vi "GetFPGABitfilePath.vi"(8 "error in (no error)":errorcluster) -> (0 "error out":errorcluster, 2 "description":string, 3 "fpga bitfile":path, 5 "found":bool)   [LabVIEW 2017, in "McsaFpgaBitfileManager.lvlib"]
uses:
  <vilib>/addons/InsightCM/Devices/Shared/Mcsa/McsaFpgaBitfileManager/McsaFpgaBitfileManager.lvlib
  <vilib>/addons/InsightCM/Utilities/GlobalConfiguration/GlobalConfiguration.lvlib
  <vilib>/addons/SystemInfoProcess/SystemInfoProcess.lvlib
  <vilib>/addons/InsightCM/Devices/Shared/Cms/CmsFpgaBitfileManager/CmsFpgaBitfileManager.lvlib
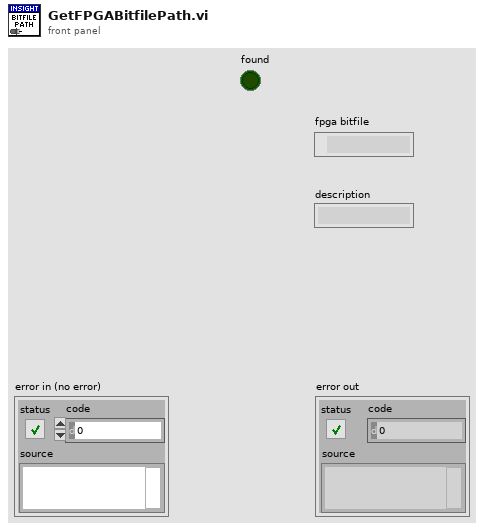
[diagram p1: front panel]
types:
  T1 = typedef "R2_Device.ctl" = cluster{"Id":string, "Name":string, "DeviceType":string, "HardwareName":string, "IpAddress":string, "HardwareInfo":T2[], "ApplicationType":string, "ApplicationVersion":string, "EquipmentIds":string[], "ConfigurationVersion":string, "State":T3, "Properties":T2[], "DataGroups":T4[], "BurstModeTrigger":T8}
  T2 = typedef "KeyValuePair.ctl" = cluster{"Key":string, "Value":string}
  T3 = typedef "DeviceState.ctl" = cluster{"Disabled":bool}
  T4 = typedef "R2_DataGroup.ctl" = cluster{"Name":string, "OperatingStates":T5[], "Properties":T2[], "EquipmentIds":string[], "AssetNodeId":string}
  T5 = typedef "OperatingState.ctl" = cluster{"Name":string, "Properties":T2[], "Triggers":T6[]}
  T6 = typedef "Trigger.ctl" = cluster{"Type":string, "Expression":string, "Conditions":T7[]}
  T7 = typedef "Condition.ctl" = cluster{"Source":string, "Type":string, "Operator":string, "CompareTo":string, "DwellSeconds":dbl}
  T8 = typedef "BurstModeTrigger.ctl" = cluster{"Trigger":T6, "SampleRate":string, "AcquisitionLength":string}
  T9 = typedef "cRIODetectHW.lvlib/SystemHW.ctl" = cluster{"controller":T10, "chassis":T10, "modules":T10[]}
  T10 = typedef "cRIODetectHW.lvlib/cRIO Product Info.ctl" = cluster{"vendorName":string, "productName":string, "serialNumber":string}
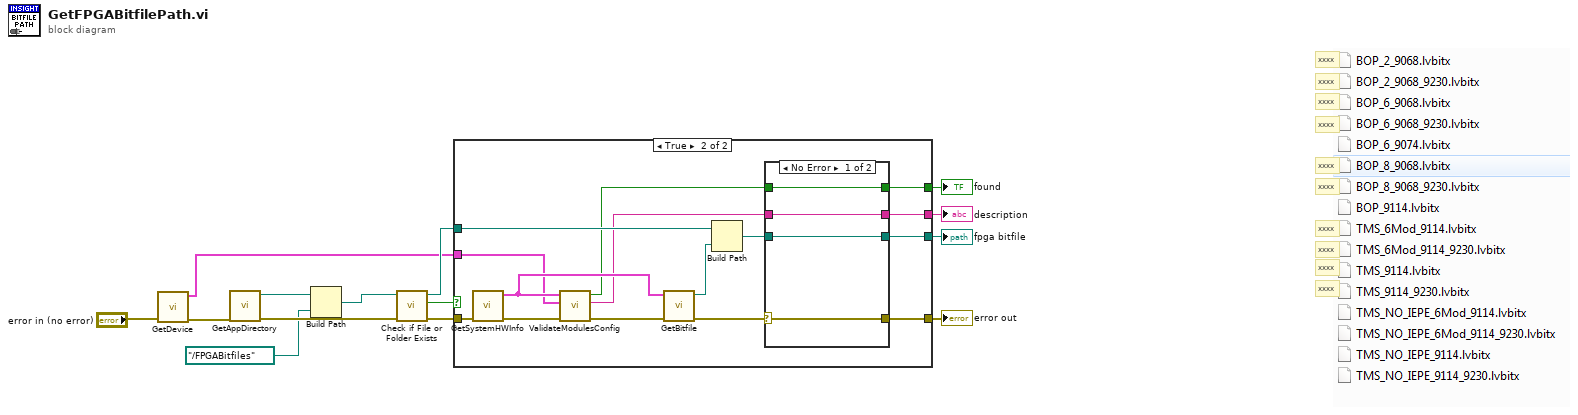
[diagram p0: block diagram]
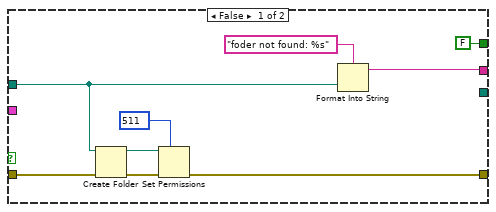
[diagram p2: hidden frame]
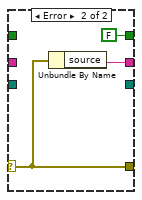
[diagram p3: hidden frame]
diagram:
  # "xxxx"
  # "xxxx"
  # "xxxx"
  # "xxxx"
  # "xxxx"
  # "xxxx"
  # "xxxx"
  # "xxxx"
  # "xxxx"
  # "xxxx"
  n1 = call <vilib>:"GetDevice.vi"("error in (no error)"="error in (no error)") -> ("error out"=w5:errorcluster, "device configuration"=w4:T1)  [unwired: 8 in, 1 out]
  n2 = call <vilib>:"GetAppDirectory.vi"("error in (no error)"=w5) -> ("error out"=w14:errorcluster, "application directory"=w13:path)  [unwired: 9 in]
  n3 = Build Path(base path=w13, name or relative path=path "../FPGABitfiles" ("application directory")) -> (appended path=w12:path)
  n4 = call <vilib>:"Check if File or Folder Exists.vi"("error in (no error)"=w14, "path"=w12) -> ("error out"=w10:errorcluster, "file or folder exists?"=w11:bool, "dup path"=w9:path)  [unwired: 7 in]
  n5 = case shown="True" w11 {
    tunnel: w10 -> [w23 w38]
    tunnel: w9 -> [w17 w34]
    tunnel: [w19 w31] -> w8
    tunnel: [_ w30] -> w7
    tunnel: w4 -> [_ w24]
    tunnel: [FALSE ("valid") w28] -> w3
    tunnel: [w15 w25] -> w1
    frame False {
      n6 = Create Folder(path (use dialog)=w17, error in=w23) -> (created path=w22:path, error out=w21:errorcluster)  [unwired: 1 in, 1 out]
      n7 = Set Permissions(7:i16 511 ("permissions"), 8:w21, 11:w22) -> (0:w19:errorcluster)  [unwired: 2 in, 1 out]
      n8 = Format Into String(format string="foder not found: %s", w17) -> (resulting string=w15:string)  [unwired: 2 in, 1 out]
    }
    frame True {
      n9 = call <vilib>:"GetSystemHWInfo.vi"("error in (no error)"=w38) -> ("error out"=w37:errorcluster, "system info"=w35:T9)  [unwired: 8 in, 1 out]
      n10 = call <vilib>:"ValidateModulesConfig.vi"("error in (no error)"=w37, "Device"=w24, "system info"=w35) -> ("error out"=w36:errorcluster, "description"=w26:string, "valid"=w27:bool)  [unwired: 6 in]
      n11 = call <vilib>:"GetBitfile.vi"("error in (no error)"=w36, "system info"=w35) -> ("error out"=w32:errorcluster, "Bitfile"=w33:path)  [unwired: 8 in]
      n12 = Build Path(base path=w34, name or relative path=w33) -> (appended path=w29:path)
      n13 = case shown="No Error" w32 {
        selector: w32 -> [w42 w45]
        tunnel: [w42 w45] -> w31
        tunnel: [w41 _] -> w30
        tunnel: w29 -> [w41 _]
        tunnel: [w40 FALSE ("valid")] -> w28
        tunnel: w27 -> [w40 _]
        tunnel: [w39 w44] -> w25
        tunnel: w26 -> [w39 _]
        frame No Error {
        }
        frame Error {
          n14 = Unbundle By Name(w45) -> ("source"=w44:string)
        }
      }
    }
  }
  "error out" <- w8
  "fpga bitfile" <- w7
  "found" <- w3
  "description" <- w1
